vi "WIP.vi"() -> ()   [LabVIEW 2018, in "LED Control Module.lvlib"]
uses:
  LED Control Module.lvlib
  Public Controls/LVS Limits.ctl
  Public Controls/LVS Settings.ctl
  Public Controls/LVS Instruments.ctl
panel:
  in  "Role":string
  in  "Username":string
  in  "LED Validation":enum32{"Validation", "Settings"}(tab)
  in  "String Control":string
  in  "History":i32(listbox)
  in  "Tester Status":string
  out "Test Status":bool
  out "Instruments":T1={"Resistor 1"=1600.0, "Resistor 2"=0.0, "Resistor 3"=0.0} caption="LED Reference Resistors" {"Resistor 3" format="%#_g ohm"; "Resistor 2" format="%#_g ohm"; "Resistor 1" format="%#f ohm"}
  in  "Exit":bool
  in  "Logout":bool
  out "Test Visualization":dbl[](graph)
  out "Part Number":string
  in  "Test Control":bool
  in  "Clear":bool
  out "LED":bool
  out "Settings":T2 {"Source V" format="%#_g V"; "VLED 3" format="%#_g V"; "VLED 2" format="%#_g V"; "VLED 1" format="%#f V"}
  out "Limits":T3 {"Wavelength" format="%#_g nm"; "Tolerance" format="%#_g %"; "Current 3" format="%#_g  mA"; "Current 2" format="%#_g  mA"; "Current 1" format="%#_g mA"}
  out "Colors [4]":cluster{u32, u32}[](array[cluster])
  # "LED Validation SYsTEM"
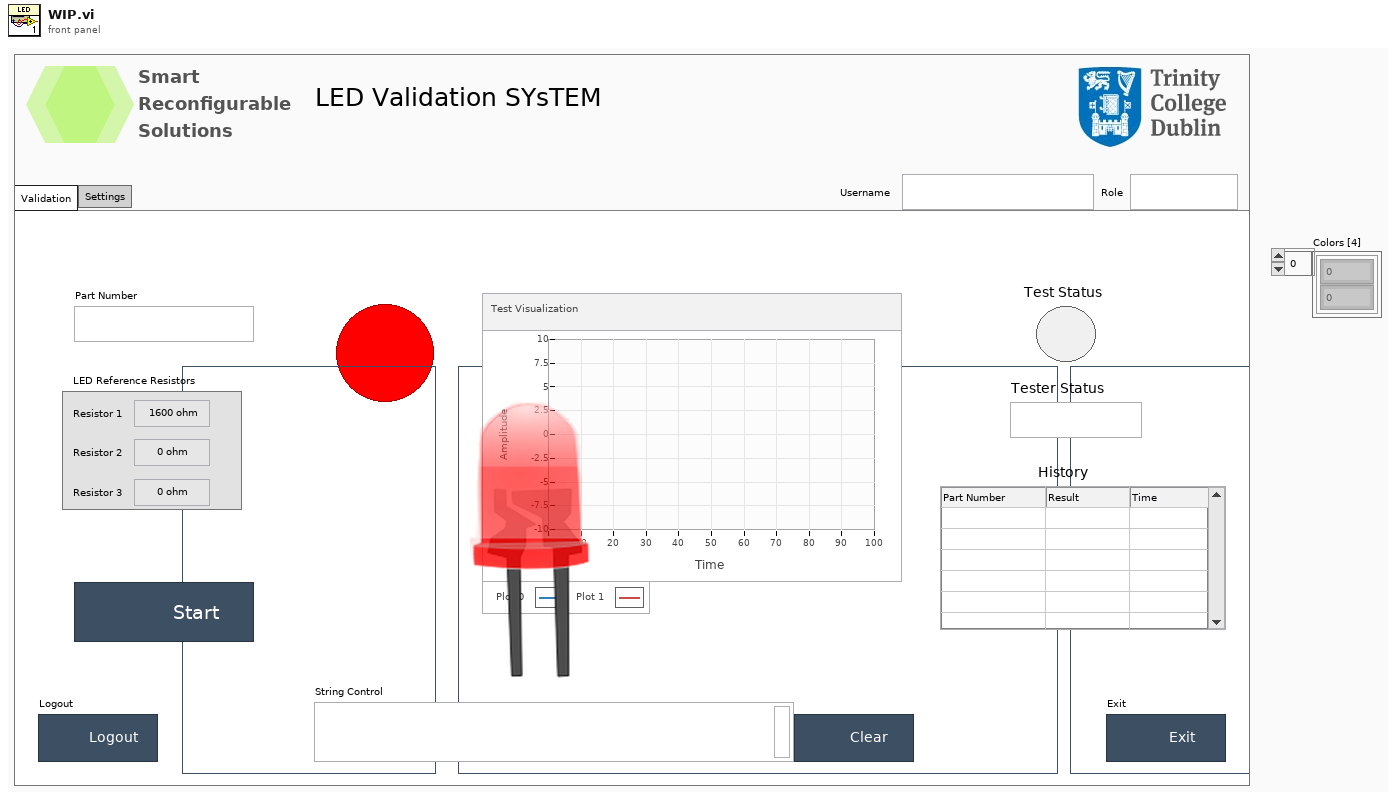
[diagram p1: front panel]
types:
  T1 = typedef "LED Control Module.lvlib/LVS Instruments.ctl" = cluster{"Resistor 1":dbl, "Resistor 2":dbl, "Resistor 3":dbl}
  T2 = typedef "LED Control Module.lvlib/LVS Settings.ctl" = cluster{"VLED 1":dbl, "VLED 2":dbl, "VLED 3":dbl, "Source V":dbl}
  T3 = typedef "LED Control Module.lvlib/LVS Limits.ctl" = cluster{"Current 1":dbl, "Current 2":dbl, "Current 3":dbl, "Tolerance":dbl, "Wavelength":dbl}
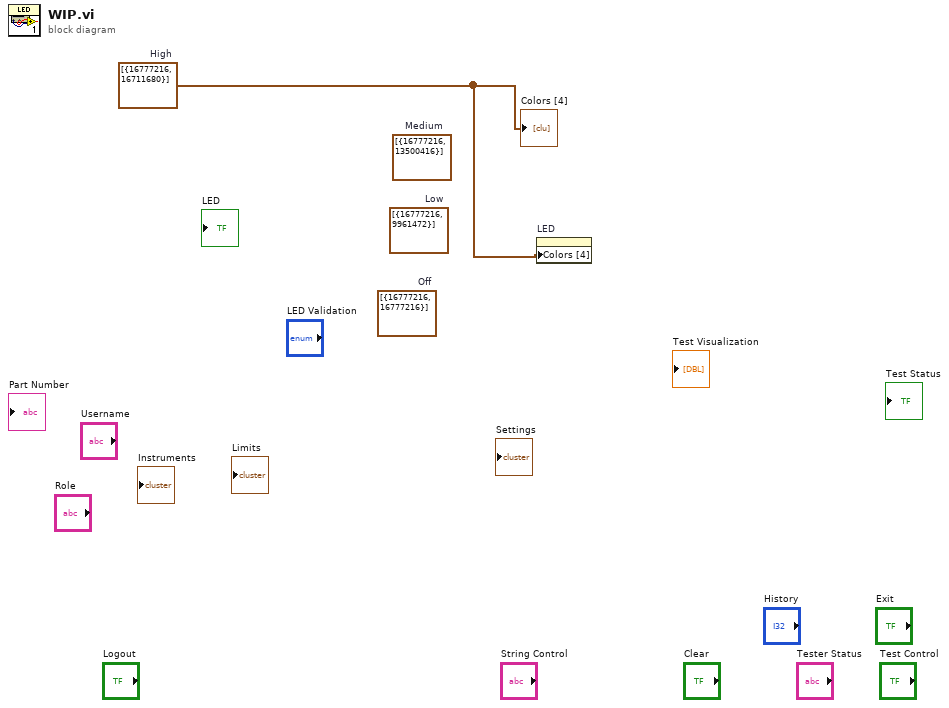
[diagram p0: block diagram]
diagram:
  (unwired) cluster{u32, u32}[] [{16777216, 16777216}]  # Off
  (unwired) cluster{u32, u32}[] [{16777216, 9961472}]  # Low
  (unwired) cluster{u32, u32}[] [{16777216, 13500416}]  # Medium
  w1 = cluster{u32, u32}[] [{16777216, 16711680}]  # High
  n1 = property on="LED" class="Bool (strict)"("Colors [4]"=w1) -> ()  [unwired: 2 in, 2 out]
  "Colors [4]" <- w1
